vi "Combine vectors with standard errors.vi"(4 "std err y":dbl, 5 "y":dbl, 6 "std err x":dbl, 7 "x":dbl) -> (1 "std err (x + y)":dbl, 2 "x+y":dbl)   [LabVIEW 2011, in "COSYLib.lvlib"]
doc: "Calculates the vectors sum of two perpendicular vectors, including standard errors"
uses:
  COSYLib.lvlib
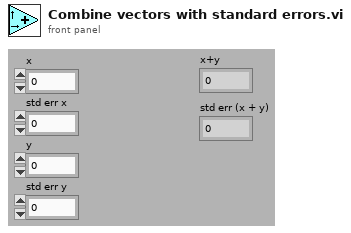
[diagram p1: front panel]
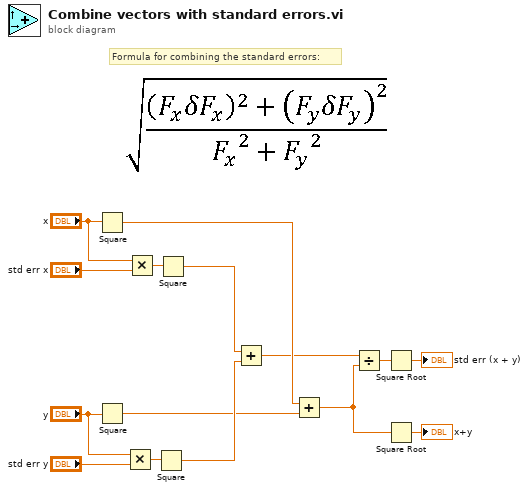
[diagram p0: block diagram]
diagram:
  # "Formula for combining the standard errors:"
  n1 = Square(x="x") -> (x^2=w7:dbl)
  n2 = Square(x="y") -> (x^2=w6:dbl)
  n3 = Multiply(x="y", y="std err y") -> (x*y=w13:dbl)
  n4 = Multiply(x="x", y="std err x") -> (x*y=w14:dbl)
  n5 = Square(x=w13) -> (x^2=w10:dbl)
  n6 = Square(x=w14) -> (x^2=w11:dbl)
  n7 = Add(x=w11, y=w10) -> (x+y=w5:dbl)
  n8 = Add(x=w7, y=w6) -> (x+y=w4:dbl)
  n9 = Divide(x=w5, y=w4) -> (x/y=w3:dbl)
  n10 = Square Root(x=w3) -> (sqrt(x)=→"std err (x + y)":dbl)
  n11 = Square Root(x=w4) -> (sqrt(x)=→"x+y":dbl)
